vi "Perform crosstalk measurement.vi"(5 "start samples/time":u32, 7 "duration":u32=1, 8 "error in":errorcluster, 9 "filter settings":T2={"Highpass filter"="DC", "Lowpass filter"="No filter", "Weighting filter"="A-weighting"}, 10 "measurement settings":T1={"Band start"=20.0, "Band stop"=20000.0, "Amplitude"=1.0, "Frequency"=1000.0, "Full scale range"=3.16}, 11 "waveforms":waveform(dbl)[](array[waveform])) -> (0 "error out":errorcluster, 3 "output cluster":T3 {"Crosstalk" format="%_6g"; "Frequency" format="%_6g"; "df" format="%_6g"; "f0" format="%_6g"; "dt" format="%_6g"; "Frequency domain" format="%_6g"; "Time domain" format="%_6g"})   [LabVIEW 2021, in "Crosstalk_Audio DAC.lvlib"]
uses:
  Crosstalk_Audio DAC.lvlib
  Measurement Results.ctl
  shared/controls/Single Tone Filter Settings.ctl
  shared/controls/Single Tone Measurement Settings.ctl
  <vilib>/addons/_NISVFA/_Shared subVIs/Common/SVL Set dB Reference (N Ch - 1 Ref).vi
  <vilib>/addons/_NISVFA/_Spectrum Processing/SVFA Unit Conversion (Complex) (N Ch).vi
  <vilib>/addons/_NISVFA/_Spectrum Processing/SVFA Unit Conversion (Complex) (1 Ch).vi
  <vilib>/addons/_NISVFA/_Shared subVIs/Common/SVL Set dB Reference (1 Ch).vi
  <vilib>/addons/_NISVFA/_Shared subVIs/Common/svc_Log View for Spectrum (1Ch).vi
  <vilib>/addons/_NISVFA/_Spectrum Processing/SVFA Unit Conversion (1 Ch).vi
  <vilib>/addons/_NISVFA/_Shared subVIs/Common/svc_Complex Datatype Defaults.vi
  <vilib>/addons/_NISVFA/_Shared subVIs/Common/SVL Set dB Reference (variant).vi
  <vilib>/addons/_NISVFA/_Shared subVIs/Common/svc_Unwrap Phase.vi
  <vilib>/addons/_NISVFA/_Shared subVIs/Common/svc_Convert Spectrum Array to dB.vi
  <vilib>/addons/_NISVFA/_Shared subVIs/Common/svc_Spectrum Units.vi
  <vilib>/addons/_NISVFA/_Spectrum Processing/subVIs/svfa_Conversion Utility (spectrum info).vi
  <vilib>/addons/_NISVFA/_Shared subVIs/Common/svc_Format Value (DBL).vi
  <vilib>/addons/_NISVFA/_Shared subVIs/Common/svc_Get Weighting Enum and Labels.vi
  <vilib>/addons/_NISVFA/_Shared subVIs/Common/svc_Engineering Units to Unit Label.vi
  <vilib>/addons/_NISVFA/_Shared subVIs/Common/svc_Surround NonAlpha String with Parentheses.vi
  <vilib>/dlg_ctls.llb/Space Constant.vi
  <vilib>/addons/_NISVFA/_Spectrum Processing/subVIs/svfa_Peak to RMS to Peak2Peak.vi
  <vilib>/addons/_NISVFA/_Spectrum Processing/subVIs/svfa_Mag to Mag2.vi
  <vilib>/addons/_NISVFA/_Spectrum Processing/subVIs/svfa_Linear to dB.vi
  <vilib>/addons/_NISVFA/_Spectrum Processing/subVIs/svfa_dBrefA to dBrefB.vi
  <vilib>/addons/_NISVFA/_Spectrum Processing/subVIs/svfa_Spectrum to Spectral Density.vi
  <vilib>/addons/_NISVFA/_Shared subVIs/Common/svc_Unit Label Lexical Class.vi
  <vilib>/addons/_NISVFA/_Shared subVIs/Common/svc_Window Parameters.vi
  <vilib>/Waveform/WDTOps.llb/WDT Get Waveform Subset DBL.vi
  <vilib>/addons/_NISVFA/_Shared subVIs/Common/svc_Caller VI Returned in Error Source.vi
  <vilib>/Analysis/4window.llb/window parameters.vi
  <vilib>/Analysis/4window.llb/Window Properties.vi
  <vilib>/Analysis/4window.llb/Window Properties by Name.vi
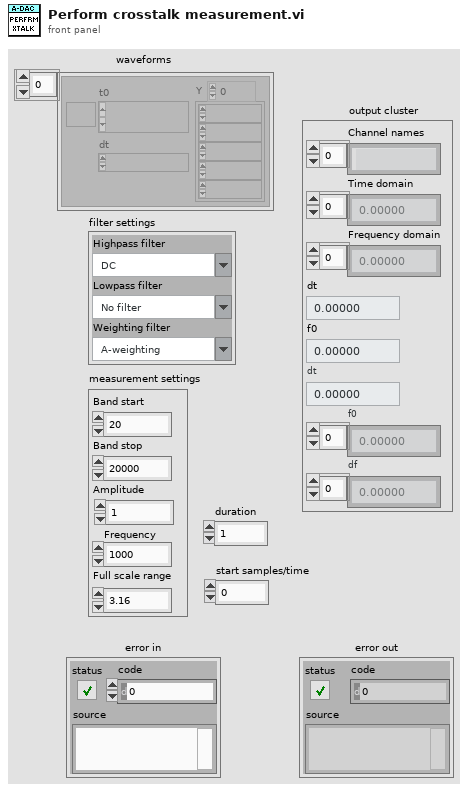
[diagram p1: front panel]
types:
  T1 = typedef "Single Tone Measurement Settings.ctl" = cluster{"Band start":dbl, "Band stop":dbl, "Amplitude":dbl, "Frequency":dbl, "Full scale range":dbl}
  T2 = typedef "Single Tone Filter Settings.ctl" = cluster{"Highpass filter":string, "Lowpass filter":string, "Weighting filter":string}
  T3 = typedef "Crosstalk_Audio DAC.lvlib/Measurement Results.ctl" = cluster{"Channel names":string[], "Time domain":dbl[], "Frequency domain":dbl[], "dt":dbl, "f0":dbl, "df":dbl, "Frequency":dbl[], "Crosstalk":dbl[]}
  T4 = cluster{"linear/dB":enum16{"no change", "linear", "dB"}, "dB reference (0: no change)":dbl, "power/magnitude":enum16{"no change", "power", "magnitude"}, "view":enum16{"no change", "rms", "peak", "peak-peak"}}
  T5 = typedef "svc_Spectrum Info.ctl" = cluster{"channel name":string, "description":string, "x-axis units":T6, "spectral info":cluster{"spectrum type":T7, "linear/dB":enum16{"linear", "dB"}, "window":u16, "window size":i32, "FFT size":i32}, "engineering units":T8, "custom label":string, "dB reference [EU]":dbl, "peak units":enum16{"rms", "peak", "peak-peak"}, "weighting filter":T9, "spectral density?":bool, "unit label":string, "spectrum skewed?":bool, "complimentary spectrum units":T10}
  T6 = typedef "svc_X-Axis Units.ctl" = u16
  T7 = typedef "svc_Spectrum Type.ctl" = enum16{"FFT Spectrum [complex]", "Amplitude [Magnitude]", "Power [Magnitude^2]", "Cross Spectrum [complex]", "Frequency Response [Complex]"}
  T8 = typedef "svc_Engineering Units Text Ring.ctl" = u16
  T9 = typedef "svc_Weighting Filter Text Ring.ctl" = u16
  T10 = typedef "svc_Complimentary Spectrum Units.ctl" = enum16{"none", "radians", "degrees", "cycles", "imaginary"}
  T11 = cluster{"complex spectrum response":cluster{"f0":dbl, "df":dbl, "complex spectrum":cdb[]}, "spectrum info":T5}
  T12 = cluster{"complex spectrum response":cluster{"f0":dbl, "df":dbl, "complex spectrum":cdb[]}, "spectrum info":T5}[]
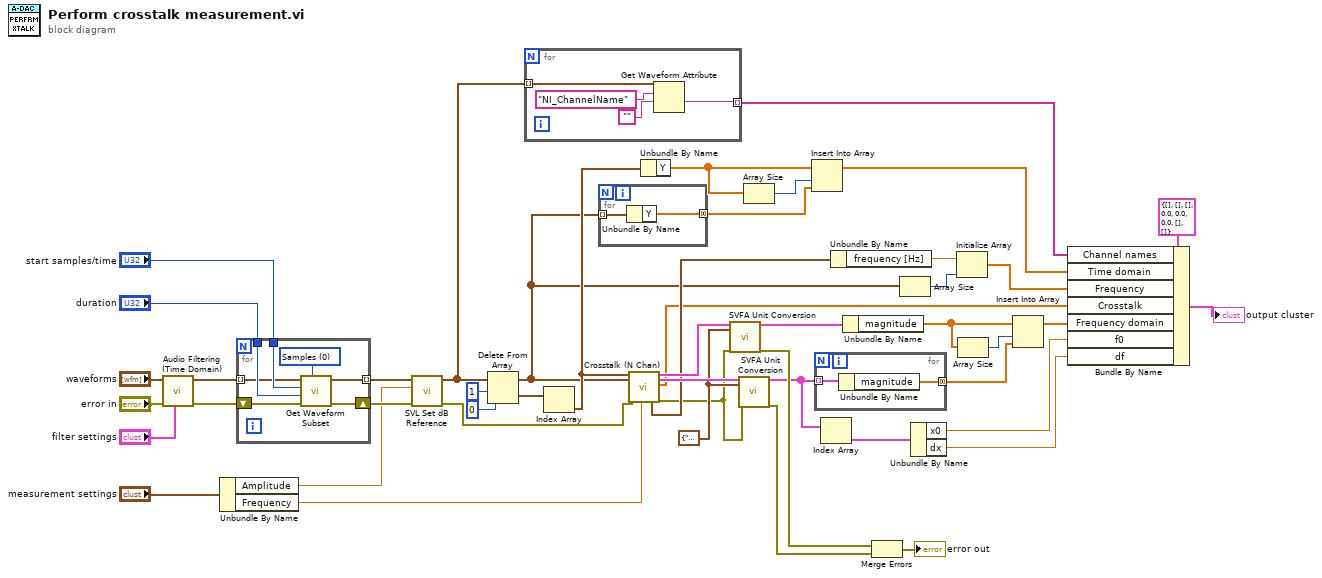
[diagram p0: block diagram]
diagram:
  w41 = T4 {"linear/dB"=enum."dB", "dB reference (0: no change)"=0.0, "power/magnitude"=enum."magnitude", "view"=enum."peak"} ("desired scaling")
  n1 = call "Audio Filtering (Time Domain).vi"("Filter settings"="filter settings", "error in"="error in", "waveforms"="waveforms") -> ("error out"=w5:errorcluster, "time domain"=w6:waveform(dbl)[])  [unwired: 7 in]
  n2 = Unbundle By Name("measurement settings") -> ("Amplitude"=w26:dbl, "Frequency"=w25:dbl)
  n3 = for {
    tunnel: [w54] -> w47 mode=indexing
    shift-right: [w51] -> w32
    shift-left: w5 -> [w52]
    tunnel: "start samples/time" -> [w50]
    tunnel: "duration" -> [w49]
    tunnel: w6 -> [w48] mode=indexing
    w53 = u16 0 items=["Samples", "Relative Time"] ("start/duration format")
    n4 = call-poly <vilib>:"Get Waveform Subset.vi"("start/duration format"=w53, "error in (no error)"=w52, "duration"=w49, "start samples/time"=w50, "waveform in"=w48) -> ("error out"=w51:errorcluster, "waveform out"=w54:waveform(dbl))  [unwired: 1 in, 2 out]
  }
  n5 = call-poly <vilib>:"SVL Set dB Reference.vi"("error in (no error)"=w32, "dB reference [EU]"=w26, "scaled signals in [EU]"=w47) -> ("error out"=w31:errorcluster, "scaled signals out [EU]"=w2:waveform(dbl)[])  [unwired: 7 in]
  n6 = Delete From Array(array=w2, length=1, index=0) -> (deleted portion=w44:waveform(dbl)[], array with subset deleted=w3:waveform(dbl)[])
  n7 = for {
    tunnel: w2 -> [w56] mode=indexing
    tunnel: [w55] -> w1 mode=indexing
    n8 = Get Waveform Attribute(5:"", 6:"NI_ChannelName" ("name"), 7:w56) -> (1:w55:string)  [unwired: 1 in, 3 out]
  }
  n9 = Index Array(array=w44) -> (element=w35:waveform(dbl))  [unwired: 1 in]
  n10 = for {
    tunnel: w3 -> [w60] mode=indexing
    tunnel: [w59] -> w14 mode=concatenating
    n11 = Unbundle By Name(w60) -> ("Y"=w59:dbl[])
  }
  n12 = call "Crosstalk (N Chan).vi"("stimulus signal"=w35, "idle channel response"=w3, "error in (no error)"=w31, "expected fundamental frequency [Hz]"=w25) -> ("detected tone stimulus"=w40:cluster{"frequency [Hz]":dbl, "amplitude":dbl}, "complex spectrum\nstimulus X"=w42:T11, "complex spectrum idle-channel response"=w43:T12, "crosstalk"=w21:dbl[], "error out"=w30:errorcluster)  [unwired: 8 in, 3 out]
  n13 = Unbundle By Name(w35) -> ("Y"=w15:dbl[])
  n14 = call-poly <vilib>:"SVFA Unit Conversion.vi"("complex spectrum"=w42, "desired scaling"=w41, "error in (no error)"=w30) -> ("converted spectrum"=w34:cluster{"x0":dbl, "dx":dbl, "magnitude":dbl[]}, "error out"=w29:errorcluster)  [unwired: 11 in, 4 out]
  n15 = call-poly <vilib>:"SVFA Unit Conversion.vi"("complex spectra"=w43, "desired scaling"=w41, "error in (no error)"=w30) -> ("converted spectra"=w13:cluster{"x0":dbl, "dx":dbl, "magnitude":dbl[]}[], "error out"=w28:errorcluster)  [unwired: 11 in, 4 out]
  n16 = Array Size(array=w15) -> (size(s)=w16:i32)
  n17 = Insert Into Array(array=w15, index=w16, new element=w14) -> (w22:dbl[])
  n18 = for {
    tunnel: w13 -> [w62] mode=indexing
    tunnel: [w61] -> w18 mode=concatenating
    n19 = Unbundle By Name(w62) -> ("magnitude"=w61:dbl[])
  }
  n20 = Index Array(array=w13) -> (element=w12:cluster{"x0":dbl, "dx":dbl, "magnitude":dbl[]})  [unwired: 1 in]
  n21 = Unbundle By Name(w40) -> ("frequency [Hz]"=w39:dbl)
  n22 = Unbundle By Name(w34) -> ("magnitude"=w20:dbl[])
  n23 = Merge Errors(w29, w28) -> (→"error out":errorcluster)
  n24 = Array Size(array=w3) -> (size(s)=w38:i32)
  n25 = Unbundle By Name(w12) -> ("x0"=w11:dbl, "dx"=w10:dbl)
  n26 = Initialize Array(w39, w38) -> (w36:dbl[])
  n27 = Array Size(array=w20) -> (size(s)=w19:i32)
  n28 = Insert Into Array(array=w20, index=w19, new element=w18) -> (w17:dbl[])
  n29 = Bundle By Name(cluster=T3 {"Channel names"=[], "Time domain"=[], "Frequency domain"=[], "dt"=0.0, "f0"=0.0, "df"=0.0, "Frequency"=[], "Crosstalk"=[]} ("measurement results"), "Channel names"=w1, "Time domain"=w22, "Frequency"=w36, "Crosstalk"=w21, "Frequency domain"=w17, "f0"=w11, "df"=w10) -> (→"output cluster":T3)
